vi "Idle Logic.vi"(10 "Logged on":bool, 11 "UUT Info":bool) -> (1 "Color Selector":T1, 2 "String":string, 3 "State":T2)   [LabVIEW 2023, in "Main.lvlib" / "Main.lvclass"]
uses:
  Project/Main.lvclass
  builds/Engine/Engine.lvlibp/Custom Controls/System Status.ctl
  Custom Controls/Color_Items.ctl
  builds/Engine/Engine.lvlibp/Project/Engine.lvclass
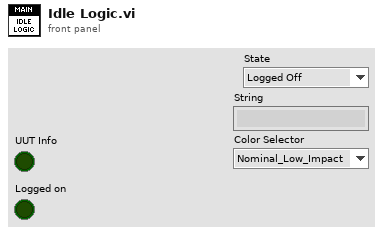
[diagram p1: front panel]
types:
  T1 = typedef "Main.lvlib/Main.lvclass/Color_Items.ctl" = enum16{"Nominal_Low_Impact", "Nominal", "User_Interaction", "Warning", "Error"}
  T2 = typedef "Engine.lvlibp/Engine.lvclass/System Status.ctl" = enum16{"Logged Off", "UUT_Info_Missing", "Idle", "Error", "Warning", "Loading", "Config", "Manual", "Automation", "Report_View", "Previous"}
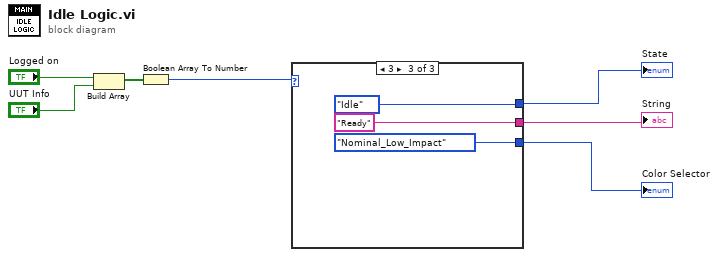
[diagram p0: block diagram]
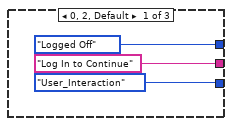
[diagram p2: hidden frame]
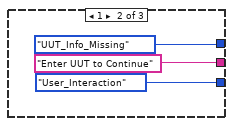
[diagram p3: hidden frame]
diagram:
  n1 = Build Array("Logged on", "UUT Info") -> (w7:bool[])
  n2 = Boolean Array To Number(Boolean array=w7) -> (number=w6:u32)
  n3 = case shown="3" w6 {
    tunnel: ["Log In to Continue" "Enter UUT to Continue" "Ready"] -> w2
    tunnel: [Color_Items."User_Interaction" ("Color Selector") Color_Items."User_Interaction" ("Color Selector") Color_Items."Nominal_Low_Impact" ("Color Selector")] -> w1
    tunnel: [System_Status."Logged Off" ("State") System_Status."UUT_Info_Missing" ("State") System_Status."Idle" ("State")] -> w3
    frame 0, 2, Default {
    }
    frame 1 {
    }
    frame 3 {
    }
  }
  "State" <- w3
  "String" <- w2
  "Color Selector" <- w1
